vi "Lin_Rohner_lab2B_question5_retest.vi"() -> ()   [LabVIEW 2019]
uses:
  <vilib>/Platform/TimedLoop/XDataNode/timing_clust.ctl
  <vilib>/Platform/TimedLoop/XDataNode/nitl_modes.ctl
  <vilib>/Platform/TimedLoop/XDataNode/wakeup.ctl
  <vilib>/Analysis/3filter.llb/Filter Passband Type.ctl
  <vilib>/DAQmx/write.llb/DAQmx Write (Analog DBL 1Chan 1Samp).vi
  <vilib>/DAQmx/read.llb/DAQmx Read (Analog DBL 1Chan 1Samp).vi
  <vilib>/DAQmx/create/channels.llb/DAQmx Create Channel (AO-Voltage-Basic).vi
  <vilib>/DAQmx/miscellaneous.llb/DAQmx Fill In Error Info.vi
  <vilib>/DAQmx/create/channels.llb/DAQmx Create Channel (AI-Voltage-Basic).vi
  <vilib>/platform/TimedLoop/XDataNode/XDataNode.xnode
  <vilib>/Platform/TimedLoop/XDataNode/XDNodeRunTimeDep.lvlib
  <vilib>/Analysis/NI_AALBase.lvlib
  <vilib>/ptbypt/NI_PtbyPt.lvlib
panel:
  out "current through shunt":dbl
  in  "data":dbl format="%0.2f"
  out "Current through Shunt":dbl(graph)
  in  "low cutoff freq for the differential voltage measurement at Shunt":dbl=0.12500000000000006 format="%0.4f"
  out "Motor Control Voltage":dbl(graph)
  in  "stop":bool
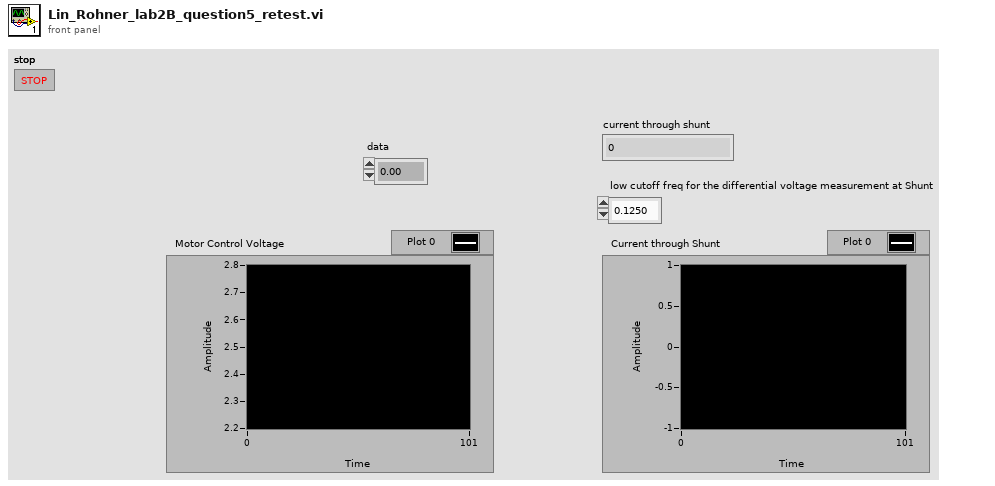
[diagram p1: front panel]
types:
  T1 = typedef "NI_AALBase.lvlib/Filter Passband Type.ctl" = enum32{"Lowpass", "Highpass", "Bandpass", "Bandstop"}
  T2 = typedef "XDNodeRunTimeDep.lvlib/timing_clust.ctl" = cluster{"Expected End [f-1]":u64, "Actual End [f-1]":u64, "Finished Late? [f-1]":bool, "Expected End [i-1]":u64, "Actual End [i-1]":u64, "Finished Late? [i-1]":bool, "Expected Start [i]":u64, "Actual Start [i]":u64, "Expected Start [f]":u64, "Actual Start [f]":u64, "Source Name":string, "Structure Name":string, "Period":i64, "Deadline":i64, "Offset":i64, "Start":i64, "Priority":i32, "Timeout":i32, "Mode":T3, "Wakeup Reason":T4, "Error":errorcluster, "Source Type":string, "Secondary Source Type":string, "Global End Time":u64, "Global Start Time":u64, "Frame Duration":u64, "Iteration Duration":u64, "Assigned CPU":i32, "I/O Scan Engine Mode":u32}
  T3 = typedef "XDNodeRunTimeDep.lvlib/nitl_modes.ctl" = enum32{"No Change", "Process missed periods, maintain original phase", "Discard missed periods, maintain original phase", "Process missed periods, ignore original phase", "Discard missed periods, ignore original phase"}
  T4 = typedef "XDNodeRunTimeDep.lvlib/wakeup.ctl" = enum32{"Normal", "Aborted", "Asynchronous wakeup", "Timing source error", "Timed loop error", "Timeout"}
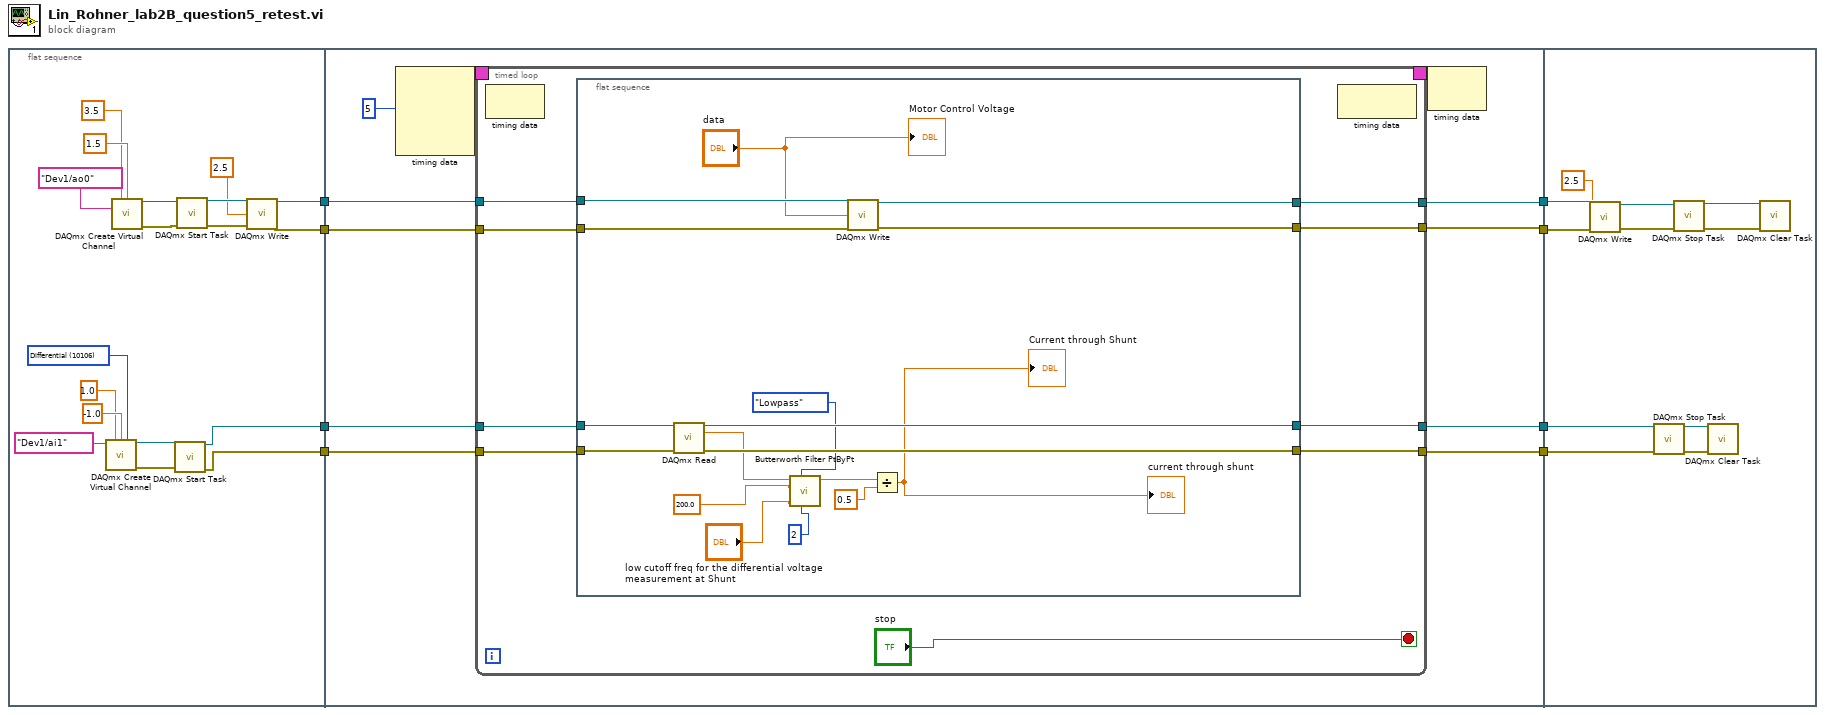
[diagram p0: block diagram]
diagram:
  n1 = flat-sequence {
    tunnel: [w24] -> w4
    tunnel: [w23] -> w3
    tunnel: [w11] -> w2
    tunnel: [w10] -> w1
    tunnel: [w35] -> w8
    tunnel: [w34] -> w7
    tunnel: [w30] -> w6
    tunnel: [w29] -> w5
    tunnel: w4 -> [w28]
    tunnel: w3 -> [w27]
    tunnel: w2 -> [w33]
    tunnel: w1 -> [w32]
    tunnel: w8 -> [w80]
    tunnel: w7 -> [w75]
    tunnel: w6 -> [w71]
    tunnel: w5 -> [w70]
    frame #0 {
      w9 = 10106 items=["Default"=-1, "RSE"=10083, "NRSE"=10078, "Differential"=10106, "Pseudodifferential"=12529] ("input terminal configuration")
      n2 = call-poly <vilib>:"DAQmx Create Virtual Channel.vi"("maximum value"=1.0, "minimum value"=-1.0, "input terminal configuration"=w9, "physical channels"=tag "Dev1/ai1") -> ("task out"=w16:refnum<k21>, "error out"=w15:errorcluster)  [unwired: 10 in]
      n3 = call-poly <vilib>:"DAQmx Create Virtual Channel.vi"("maximum value"=3.5, "minimum value"=1.5, "physical channels"=tag "Dev1/ao0") -> ("task out"=w26:refnum<k21>, "error out"=w22:errorcluster)  [unwired: 11 in]
      n4 = call <vilib>:"DAQmx Start Task.vi"("task/channels in"=w16, "error in"=w15) -> ("task out"=w11:refnum<k21>, "error out"=w10:errorcluster)  [unwired: 12 in]
      n5 = call <vilib>:"DAQmx Start Task.vi"("task/channels in"=w26, "error in"=w22) -> ("task out"=w25:refnum<k21>, "error out"=w21:errorcluster)  [unwired: 12 in]
      n6 = call-poly <vilib>:"DAQmx Write.vi"("task/channels in"=w25, "data"=2.5, "error in"=w21) -> ("task out"=w24:refnum<k21>, "error out"=w23:errorcluster)  [unwired: 10 in, 1 out]
    }
    frame #1 {
      n7 = node-c288(i64 5 ("Period")) -> (w37:T2)  [unwired: 3 in]
      n8 = timed-loop {
        timing: w37 -> [_]
        timing-out: [_] -> w36
        tunnel: w28 -> [w46]
        tunnel: w27 -> [w44]
        tunnel: [w45] -> w35
        tunnel: [w43] -> w34
        tunnel: w33 -> [w42]
        tunnel: w32 -> [w41]
        tunnel: [w40] -> w30
        tunnel: [w39] -> w29
        stop <- "stop" stop-if-true
        n9 = node-c288() -> ()  [unwired: 1 in, 1 out]
        n10 = flat-sequence {
          tunnel: [w60] -> w39
          tunnel: [w61] -> w40
          tunnel: [w62] -> w43
          tunnel: [w63] -> w45
          tunnel: w41 -> [w50]
          tunnel: w42 -> [w51]
          tunnel: w44 -> [w48]
          tunnel: w46 -> [w49]
          frame #0 {
            n11 = call-poly <vilib>:"DAQmx Read.vi"("task/channels in"=w51, "error in"=w50) -> ("task out"=w61:refnum<k21>, "data"=w53:dbl, "error out"=w60:errorcluster)  [unwired: 11 in]
            n12 = call <vilib>:"Butterworth Filter PtByPt.vi"("order"=2, "filter type"=Filter_Passband_Type."Lowpass", "low cutoff freq: fl"="low cutoff freq for the differential voltage measurement at Shunt", "sampling freq: fs"=200.0, "x"=w53) -> ("Filtered x"=w57:dbl)  [unwired: 4 in, 1 out]
            n13 = call-poly <vilib>:"DAQmx Write.vi"("task/channels in"=w49, "data"="data", "error in"=w48) -> ("task out"=w63:refnum<k21>, "error out"=w62:errorcluster)  [unwired: 10 in, 1 out]
            n14 = Divide(x=w57, y=0.5) -> (x/y=→"Current through Shunt" →"current through shunt":dbl)
            "Motor Control Voltage" <- "data"
          }
        }
        n15 = node-c288() -> ()  [unwired: 1 in, 1 out]
      }
      n16 = node-c288(w36) -> ()  [unwired: 1 out]
    }
    frame #2 {
      n17 = call-poly <vilib>:"DAQmx Write.vi"("task/channels in"=w80, "data"=2.5, "error in"=w75) -> ("task out"=w79:refnum<k21>, "error out"=w76:errorcluster)  [unwired: 10 in, 1 out]
      n18 = call <vilib>:"DAQmx Stop Task.vi"("task/channels in"=w71, "error in"=w70) -> ("task out"=w73:refnum<k21>, "error out"=w72:errorcluster)  [unwired: 12 in]
      n19 = call <vilib>:"DAQmx Stop Task.vi"("task/channels in"=w79, "error in"=w76) -> ("task out"=w78:refnum<k21>, "error out"=w77:errorcluster)  [unwired: 12 in]
      n20 = call <vilib>:"DAQmx Clear Task.vi"("task in"=w73, "error in"=w72) -> ()  [unwired: 13 in, 1 out]
      n21 = call <vilib>:"DAQmx Clear Task.vi"("task in"=w78, "error in"=w77) -> ()  [unwired: 13 in, 1 out]
    }
  }
